vi "GT Buf Synch Prf Pos.vi"(6 "fifo":i16, 7 "profile":i16, 8 "error in (no error)":errorcluster caption="错误输入（无错误）", 9 "encoder":i16, 10 "crd":i16, 11 "cardNum":i16) -> (0 "error out":errorcluster caption="错误输出", 3 "function return":i16)   [LabVIEW 2020, in "gts.lvlib"]
doc: "GT_API GT_BufSynchPrfPos(short cardNum,short crd,short encoder,short profile,short fifo=0);"
uses:
  gts.lvlib
  dll/32bit/multi_card/gts.dll
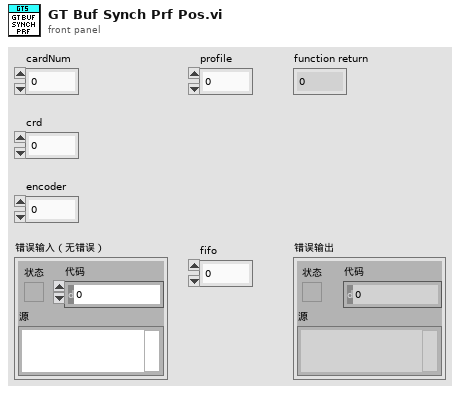
[diagram p1: front panel]
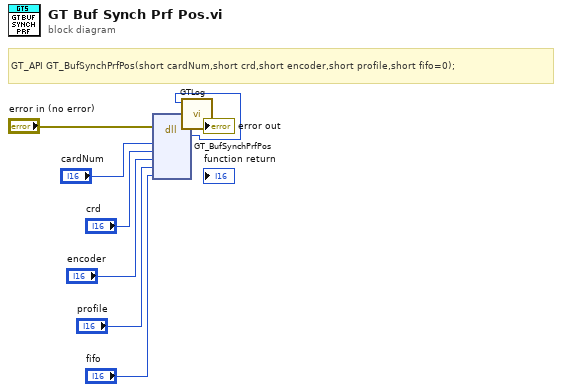
[diagram p0: block diagram]
diagram:
  # "GT_API GT_BufSynchPrfPos(short cardNum,short crd,short encoder,short profile,short fifo=0);"
  n1 = dll-call lib="C:/1228/dll/32bit/multi_card/gts.dll" fn="GT_BufSynchPrfPos"(error in="error in (no error)", "cardNum"="cardNum", "crd"="crd", "encoder"="encoder", "profile"="profile", "fifo"="fifo") -> (error out=w3:errorcluster, w1:i16)  [unwired: 7 in, 1 out]
  n2 = call "GTLog.vi"("error in (no error)"=w3, "Numeric"=w1) -> ("error out"=→"error out":errorcluster)  [unwired: 9 in]
